vi "Get Theme Mode.vi"(8 "error in":errorcluster, 11 "Theme Config in":refnum<class "Theme Config.lvclass">) -> (0 "error out":errorcluster, 2 "Theme Mode":u16(ring) items=["Light Theme", "Light Medium Contrast", "Light High Contrast", "Dark Theme", "Dark Medium Contrast", "Dark High Constrast"], 3 "Theme Config out":refnum<class "Theme Config.lvclass">)   [LabVIEW 2021, in "Theme Config.lvclass"]
doc: "data member access:\n\nget the theme mode\n\n<b>Code Developed By:</b> +\nDaniel Coons +\nTechnology Service Corporation +\nwww.tsc.com/atcs"
uses:
  Theme Config.lvclass
  Theme Config.lvclass/Theme Config.ctl
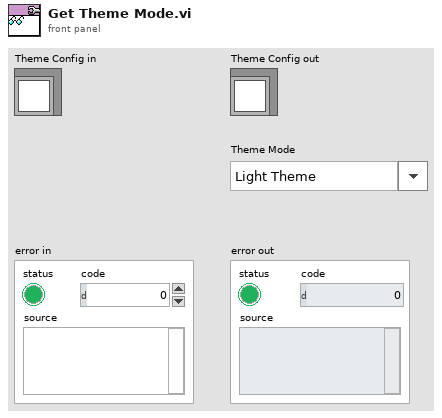
[diagram p1: front panel]
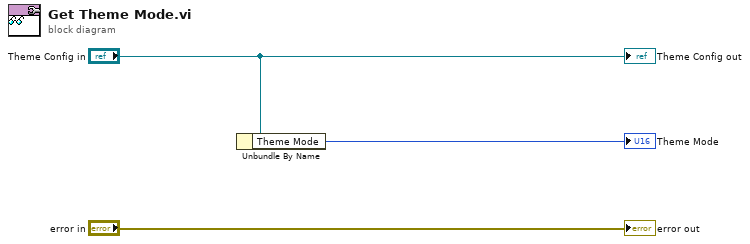
[diagram p0: block diagram]
diagram:
  n1 = Unbundle By Name("Theme Config in") -> ("Theme Mode"=→"Theme Mode":u16)
  "error out" <- "error in"
  "Theme Config out" <- "Theme Config in"
